vi "Avocent_build_command_ON.vi"(8 "error in":errorcluster, 11 "Set switches":bool[](array[boolean])=[FALSE, TRUE, TRUE, FALSE, TRUE, TRUE, FALSE, FALSE, TRUE, FALSE, TRUE, TRUE, TRUE, TRUE, TRUE, TRUE, FALSE, FALSE, FALSE, FALSE, FALSE, FALSE, FALSE, FALSE, FALSE, FALSE, FALSE, FALSE, FALSE, FALSE, FALSE, FALSE] caption="Set Switches") -> (0 "error out":errorcluster, 3 "HTTP command":string="/1?3=admin,1234,0110110010111111,")   [LabVIEW 2013]
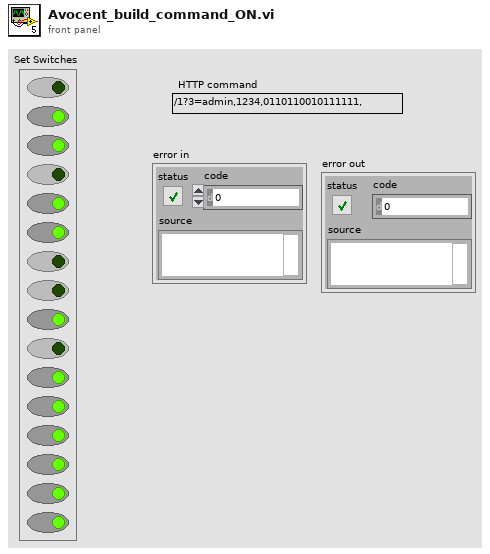
[diagram p1: front panel]
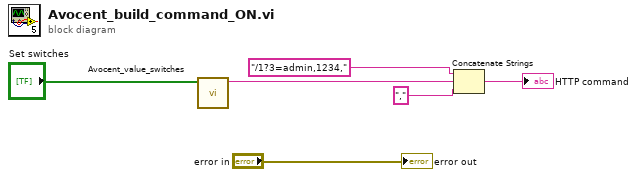
[diagram p0: block diagram]
diagram:
  n1 = call "Avocent_value_switches.vi"("Power indicator 2"="Set switches") -> ("spreadsheet string"=w4:string)  [unwired: 10 in]
  n2 = Concatenate Strings("/1?3=admin,1234," ("Command"), w4, "," ("Command")) -> (→"HTTP command":string)
  "error out" <- "error in"
